vi "WhileLoopAsForLoop.vi"() -> ()   [LabVIEW 2025]
panel:
  out "Iterations Completed":dbl
  in  "stop":bool
  in  "limit":dbl
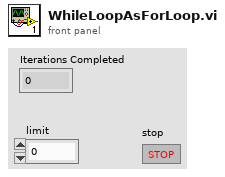
[diagram p1: front panel]
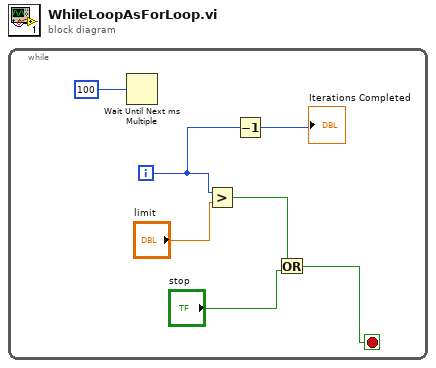
[diagram p0: block diagram]
diagram:
  n1 = while {
    i -> [w2]
    stop <- w4 stop-if-true
    n2 = Wait Until Next ms Multiple(millisecond multiple=100) -> ()  [unwired: 1 out]
    n3 = Greater?(x=w2, y="limit") -> (0:w5:bool)
    n4 = Decrement(x=w2) -> (x-1=→"Iterations Completed":i32)
    n5 = Or(x=w5, y="stop") -> (x .or. y?=w4:bool)
  }
